vi "CODMn启动命令 (子VI).vi"(11 "启动测量模式":T1) -> ()   [LabVIEW 2016, in "斯坦道CODMn.lvlib"]
uses:
  <vilib>/Plasmionique/MB Master/MB_Master_Serial/MB_Master_Serial.lvclass
  C:/Program Files (x86)/National Instruments/LabVIEW 2016/vi.lib/Plasmionique/MB Master/MB_Master/MB_Master.lvclass
  <vilib>/Plasmionique/MB Master/MB Master.lvlib
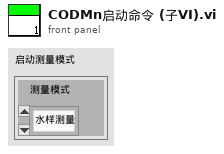
[diagram p1: front panel]
types:
  T1 = cluster{"测量模式":enum16{"水样测量", "标样核查", "零点核查", "加标回收", "平行样", "校零", "校标"}}
  T2 = cluster{"baud rate (bps)":u32, "stop bits":u16, "parity":u16, "flow control":u16, "timeout":u32, "retries":i32}
  T3 = enum16{"水样测量", "标样核查", "零点核查", "加标回收", "平行样", "校零", "校标"}
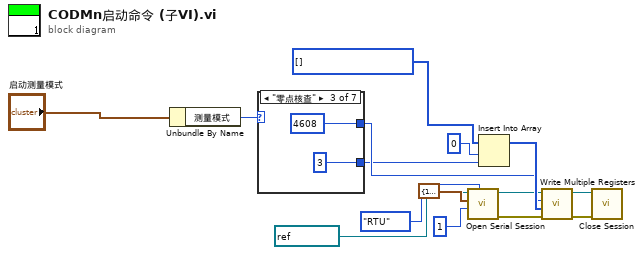
[diagram p0: block diagram]
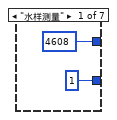
[diagram p2: hidden frame]
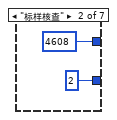
[diagram p3: hidden frame]
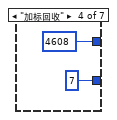
[diagram p4: hidden frame]
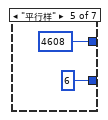
[diagram p5: hidden frame]
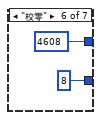
[diagram p6: hidden frame]
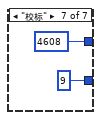
[diagram p7: hidden frame]
diagram:
  n1 = Unbundle By Name("启动测量模式") -> ("测量模式"=w7:T3)
  n2 = case shown="\"零点核查\"" w7 {
    tunnel: [u16 4608 ("address") u16 4608 ("address") u16 4608 ("address") u16 4608 ("address") u16 4608 ("address") u16 4608 ("address") u16 4608 ("address")] -> w12
    tunnel: [u16 1 ("address") u16 2 ("address") u16 3 ("address") u16 7 ("address") u16 6 ("address") u16 8 ("address") u16 9 ("address")] -> w5
    frame "水样测量" {
    }
    frame "标样核查" {
    }
    frame "零点核查" {
    }
    frame "加标回收" {
    }
    frame "平行样" {
    }
    frame "校零" {
    }
    frame "校标" {
    }
  }
  n3 = call <vilib>:"Open Serial Session.vi"("Mode (RTU)"=enum16{"RTU", "ASCII"}."RTU", "Slave ID"=u8 1, "Serial Config"=T2 {"baud rate (bps)"=115200, "stop bits"=10, "parity"=0, "flow control"=0, "timeout"=1000, "retries"=1}, "VISA Resource"=refnum<visa-resource-name> "COM3") -> ("Error out"=w15:errorcluster, "MB_Serial session"=w1:refnum<class "MB_Master_Serial.lvclass">)  [unwired: 6 in]
  n4 = Insert Into Array(array=u16[] [] ("values"), index=0 ("索引"), new element=w5) -> (w13:u16[])
  n5 = call <vilib>:"Write Multiple Registers.vi"("error in (no error)"=w15, "values"=w13, "starting address"=w12, "MB session in"=w1) -> ("error out"=w14:errorcluster, "MB session out"=w2:refnum<class "MB_Master_Serial.lvclass">)  [unwired: 6 in]
  n6 = call-dynamic "Close Session.vi"("error in (no error)"=w14, "MB_Serial session"=w2) -> ()  [unwired: 9 in, 1 out]
